vi "Get Data Version String.vi"(8 "error in (no error)":errorcluster, 11 "Configuration in":refnum<class "Configuration.lvclass">) -> (0 "error out":errorcluster, 2 "data version":string, 3 "Configuration out":refnum<class "Configuration.lvclass">)   [LabVIEW 2017, in "DSF Core.lvlib" / "Configuration.lvclass"]
uses:
  Configuration.lvclass
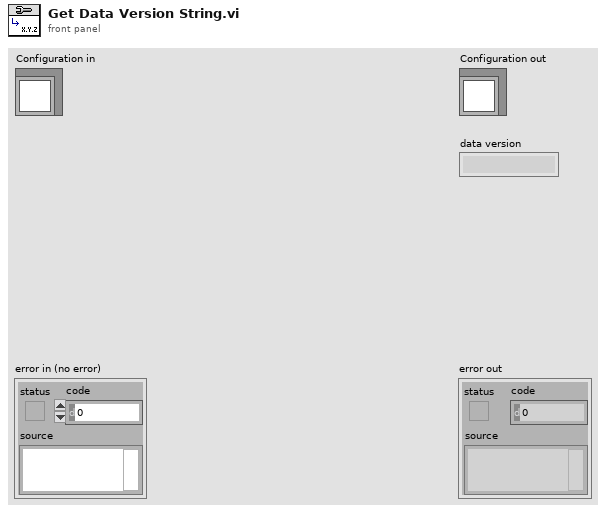
[diagram p1: front panel]
types:
  T1 = typedef "DSF Core.lvlib/DSF Version Info.ctl" = cluster{"major":u32, "minor":u32, "fix":u32, "build":string}
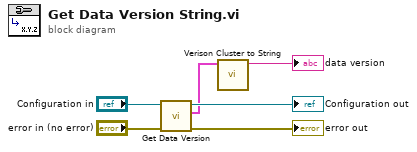
[diagram p0: block diagram]
diagram:
  n1 = call-dynamic "Get Data Version.vi"("error in (no error)"="error in (no error)", "Configuration in"="Configuration in") -> ("error out"=→"error out":errorcluster, "data version"=w3:T1, "Configuration out"=→"Configuration out":refnum<class "Configuration.lvclass">)  [unwired: 7 in]
  n2 = call "Verison Cluster to String.vi"("version"=w3) -> ("version string"=→"data version":string)  [unwired: 10 in]
